vi "getTimeMov.vi"(9 "Yf·s":dbl, 10 "传感器索引":i32=1, 11 "不包含头的全量数组数据":string[][](array[string])) -> (3 "时漂":dbl)   [LabVIEW 2017]
panel:
  # "计算时漂"
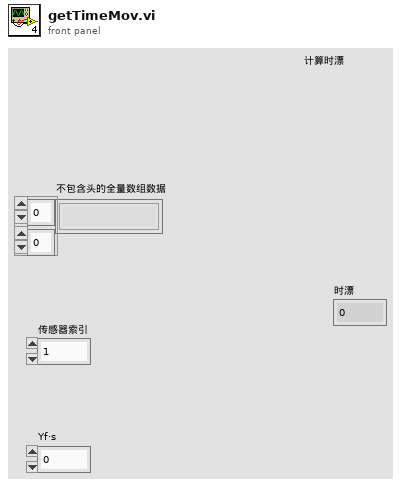
[diagram p1: front panel]
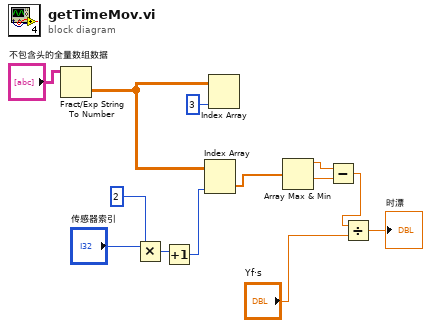
[diagram p0: block diagram]
diagram:
  n1 = Fract/Exp String To Number(string="不包含头的全量数组数据") -> (number=w1:dbl[][])  [unwired: 3 in, 1 out]
  n2 = Multiply(x="传感器索引", y=2) -> (x*y=w10:i32)
  n3 = Increment(x=w10) -> (x+1=w9:i32)
  n4 = Index Array(array=w1, index (col)=w9) -> (element=w8:dbl[])  [unwired: 1 in]
  n5 = Index Array(array=w1, index (col)=3 ("禁用的索引 (列)")) -> ()  [unwired: 1 in, 1 out]
  n6 = Array Max & Min(array=w8) -> (max value=w6:dbl, min value=w7:dbl)  [unwired: 2 out]
  n7 = Subtract(x=w6, y=w7) -> (x-y=w5:dbl)
  n8 = Divide(x=w5, y="Yf·s") -> (x/y=→"时漂":dbl)
